vi "PH_Stepmotor_BaseClass.START Axes PSDB THREAD.vi"(0 "VI in":refnum<vi>, 5 "error in (no error)":errorcluster) -> (14 "VI out":refnum<vi>, 19 "error out":errorcluster)   [LabVIEW 2014, in "PH_Stepmotor_BaseClass.lvlib"]
uses:
  PH_Stepmotor_BaseClass.lvlib
  CS_Core/CSSystem/CSSystemLib/CSSystemLib.lvlib
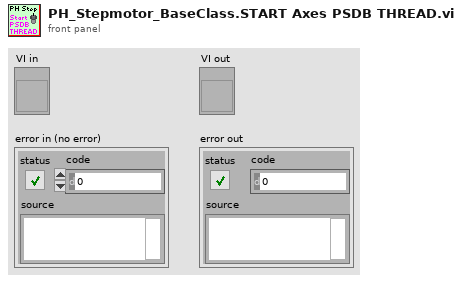
[diagram p1: front panel]
types:
  T1 = typedef "PH_Stepmotor_BaseClass.lvlib/PH_Stepmotor_BaseClass.i attribute.ctl" = cluster{"Device Error":errorcluster, "Axes PSDB Thread":cluster{"Ref":refnum<vi>, "Q-Ref":refnum<queue>, "Data Status":T2}, "Axes":T3[], "Axes PSDB Infos":cluster{"GUI Name":string, "PSDB Instance ID":i32, "PSDB Status Service ID":i32, "Axis":i32, "Class":string}[], "GUI Refs":T8}
  T2 = typedef "PH_PSDBWriter.lvlib/PH_PSDBWriter.Data Status.ctl" = i16
  T3 = typedef "PH_Stepmotor_BaseClass.lvlib/PH_Stepmotor_BaseClass.Axis Attributes.ctl" = cluster{"Settings":T4, "Endswitch?":bool, "DIM Service IDs":T6, "Activity":T7, "Configured?":bool, "Position":cluster{"Current":i32, "Target":i32}, "Position to set":cluster{"New?":bool, "Wanted":i32}, "Stop?":bool, "Reset?":bool, "Move?":bool, "Nothing connected?":bool}
  T4 = typedef "PH_Stepmotor_BaseClass.lvlib/PH_Stepmotor_BaseClass.Axis Settings.ctl" = cluster{"Sign change":bool, "Width":dbl, "Calibration":dbl, "Unit":string, "Motor Type":T5, "Unit Width":string, "Unit CF":string}
  T5 = typedef "PH_Stepmotor_BaseClass.lvlib/PH_Stepmotor_BaseClass.Motor Type.ctl" = enum16{"Unspecific", "OWIS 49.120.2633", "OWIS 49.060.1033", "OWIS 43.040.2558", "Diamond Motion 2200 series", "OWIS 49.120.266B.MV6", "Calorimeter", "Linear Stage 1", "MICOS VT-80", "MICOS VT-80 S", "Standa Rotstage nt0.95A", "PUF RA 320.200", "PUF RA 800.200", "PUF RA 800.400", "PUF RA 400.50", "1324.nn.800.50", "1324.n9c.800.50", "1324.nn.320.200", "1324.nn.400.200", "1324.nn.800.200", "1324.nn.400.50", "1324.8c9c.800.50", "1324.8c9c.400.200"}
  T6 = typedef "PH_Stepmotor_BaseClass.lvlib/PH_Stepmotor_BaseClass.Axis DIM Service IDs.ctl" = cluster{"Settings":i32, "Information":i32}
  T7 = typedef "PH_Stepmotor_BaseClass.lvlib/PH_Stepmotor_BaseClass.Axis Activity.ctl" = enum16{"No Information", "stopped", "running", "Failure", "Alarm", "stopped at backward ES", "stopped at foreward ES"}
  T8 = typedef "PH_Stepmotor_BaseClass.lvlib/PH_Stepmotor_BaseClass.GUI Refs.ctl" = cluster{"Axes Configuration":refnum<vi>, "Device Error":refnum<vi>, "Axes PSDB Infos":refnum<vi>}
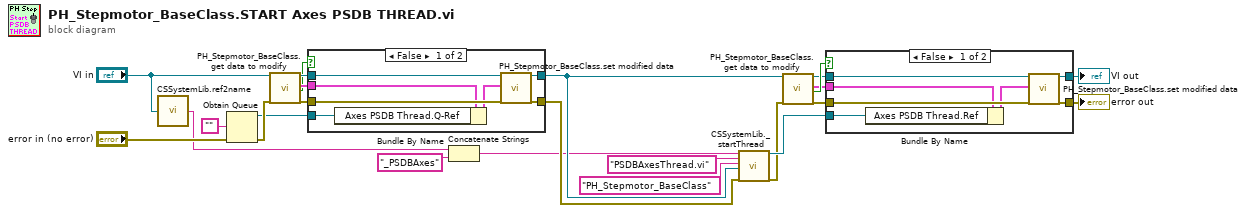
[diagram p0: block diagram]
diagram:
  n1 = call "CSSystemLib.ref2name.vi"("obj refnum"="VI in") -> ("name"=w3:string)
  n2 = Obtain Queue(element data type="", error in (no error)="error in (no error)") -> (queue out=w22:refnum<queue>, error out=w24:errorcluster)  [unwired: 3 in, 1 out]
  n3 = call "PH_Stepmotor_BaseClass.get data to modify.vi"("i ref in"="VI in", "error in (no error)"=w24) -> ("i ref out"=w19:refnum<vi>, "i attribute"=w17:T1, "timed out"=w16:bool, "error out"=w18:errorcluster)  [unwired: 14 in]
  n4 = case shown="False" w16 {
    tunnel: w19 -> [w31 w33]
    tunnel: [w30 w33] -> w21
    tunnel: w18 -> [w29 w32]
    tunnel: [w28 w32] -> w5
    tunnel: w17 -> [w27 _]
    tunnel: w22 -> [w25 _]
    frame False {
      n5 = Bundle By Name(cluster=w27, "Axes PSDB Thread.Q-Ref"=w25) -> (w26:T1)
      n6 = call "PH_Stepmotor_BaseClass.set modified data.vi"("i ref in"=w31, "i attribute"=w26, "error in (no error)"=w29) -> ("i ref out"=w30:refnum<vi>, "error out"=w28:errorcluster)  [unwired: 15 in]
    }
    frame True {
    }
  }
  n7 = Concatenate Strings(w3, "_PSDBAxes" ("thread name")) -> (w1:string)
  n8 = call "CSSystemLib._startThread.vi"("thread name"=w1, "template name"="PSDBAxesThread.vi", "Class"="PH_Stepmotor_BaseClass", "object ref"=w21, "error in (no error)"=w5) -> ("thread ref"=w14:refnum<vi>, "error out"=w11:errorcluster)  [unwired: 12 in, 1 out]
  n9 = call "PH_Stepmotor_BaseClass.get data to modify.vi"("i ref in"=w21, "error in (no error)"=w11) -> ("i ref out"=w8:refnum<vi>, "i attribute"=w13:T1, "timed out"=w15:bool, "error out"=w10:errorcluster)  [unwired: 14 in]
  n10 = case shown="False" w15 {
    tunnel: w8 -> [w40 w42]
    tunnel: [w39 w42] -> w9
    tunnel: w10 -> [w38 w41]
    tunnel: [w37 w41] -> w12
    tunnel: w13 -> [w36 _]
    tunnel: w14 -> [w34 _]
    frame False {
      n11 = Bundle By Name(cluster=w36, "Axes PSDB Thread.Ref"=w34) -> (w35:T1)
      n12 = call "PH_Stepmotor_BaseClass.set modified data.vi"("i ref in"=w40, "i attribute"=w35, "error in (no error)"=w38) -> ("i ref out"=w39:refnum<vi>, "error out"=w37:errorcluster)  [unwired: 15 in]
    }
    frame True {
    }
  }
  "error out" <- w12
  "VI out" <- w9
